vi "hDACsubtract2013.vi"(0 "FPGA VI Reference In":refnum<k20>, 7 "Ranges":u8[](array[numeric]), 11 "error in":errorcluster) -> (4 "FPGA VI Reference Out":refnum<k20>, 14 "DACbits":u16[](array[numeric]), 15 "error out":errorcluster)   [LabVIEW 2014]
doc: "Führt einen Abgleich des Offsets mit den zuvor eingelesenen Daten aus.\nAuflösung ist bei Brücke als Referenz 2,5mV ; bei 2,5V als Referenz 1,25 mV."
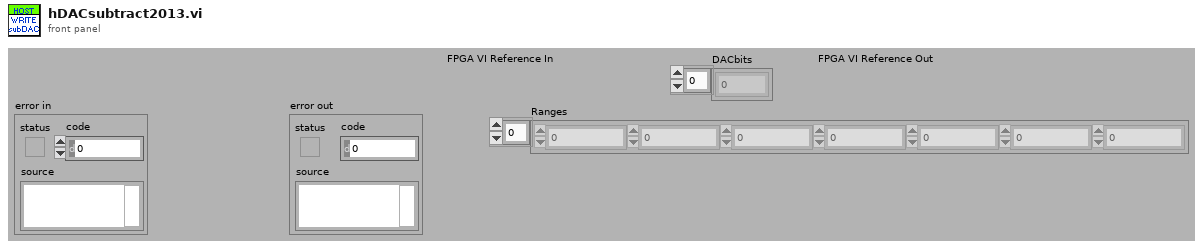
[diagram p1: front panel]
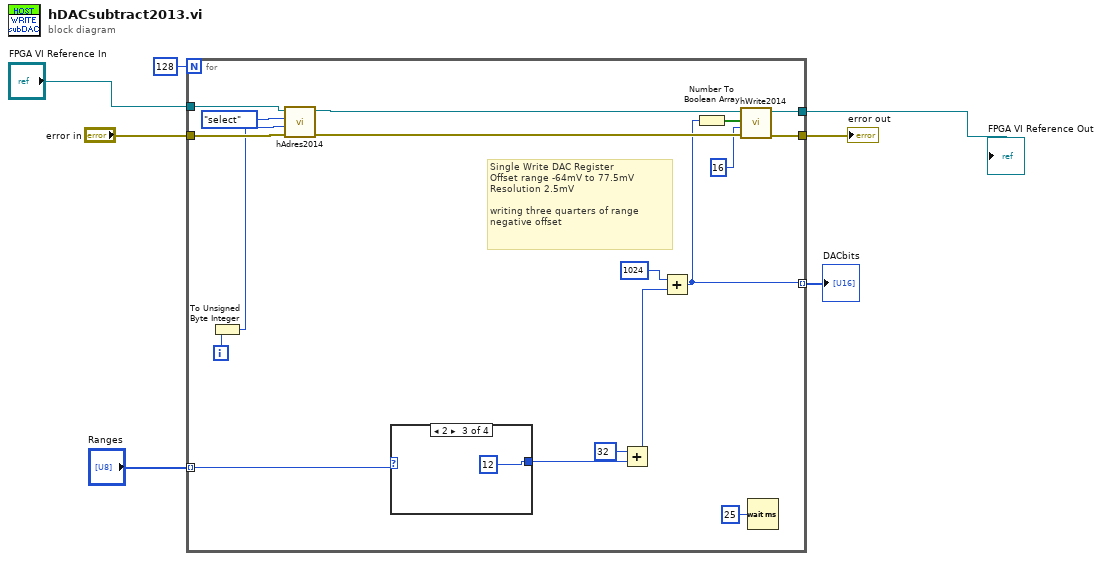
[diagram p0: block diagram]
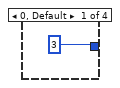
[diagram p2: hidden frame]
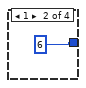
[diagram p3: hidden frame]
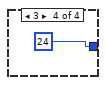
[diagram p4: hidden frame]
diagram:
  n1 = for {
    N: 128 -> [_]
    tunnel: "Ranges" -> [w11] mode=indexing
    tunnel: "error in" -> [w18]
    tunnel: [w20] -> w3
    tunnel: [w21] -> w7
    tunnel: "FPGA VI Reference In" -> [w14]
    tunnel: [w8] -> w5 mode=indexing
    i -> [w22]
    # "Single Write DAC Register\nOffset range -64mV to 77.5mV\nResolution 2.5mV\n\nwriting three quarters of range negative offset"
    n2 = To Unsigned Byte Integer(number=w22) -> (unsigned 8bit integer=w17:u8)
    n3 = call "hAdres2014.vi"("error in"=w18, "Kanal#"=w17, "AdressMode"=enum16{"select", "oben", "unten", "keinen"}."select", "FPGA VI Reference In"=w14) -> ("error out"=w15:errorcluster, "FPGA VI Reference Out"=w16:refnum<k20>)  [unwired: 2 in]
    n4 = case shown="2" w11 {
      tunnel: [u8 3 u8 6 u8 12 u8 24] -> w9
      frame 0, Default {
      }
      frame 1 {
      }
      frame 2 {
      }
      frame 3 {
      }
    }
    n5 = Add(x=u8 32, y=w9) -> (x+y=w10:u8)
    n6 = Add(x=u16 1024, y=w10) -> (x+y=w8:u16)
    n7 = Number To Boolean Array(number=w8) -> (Boolean array=w13:bool[])
    n8 = call "hWrite2014.vi"("error in"=w15, "nbit"=u8 16, "Data"=w13, "FPGA VI Reference In"=w16) -> ("error out"=w21:errorcluster, "FPGA VI Reference Out"=w20:refnum<k20>)  [unwired: 1 in, 1 out]
    n9 = Wait (ms)(milliseconds to wait=u8 25 ("Count(uSec)")) -> ()  [unwired: 1 out]
  }
  "error out" <- w7
  "DACbits" <- w5
  "FPGA VI Reference Out" <- w3
